vi "Read Aweight.vi"(8 "error in (no error)":errorcluster, 11 "Noise in":refnum<class "Noise.lvclass">) -> (0 "error out":errorcluster, 2 "Aweight":bool, 3 "Noise out":refnum<class "Noise.lvclass">)   [LabVIEW 2020, in "Noise.lvclass"]
uses:
  Noise.lvclass
  Noise.lvclass/Noise.ctl
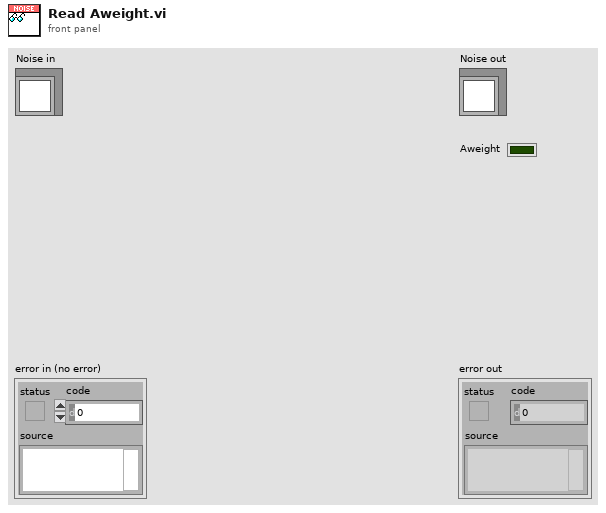
[diagram p1: front panel]
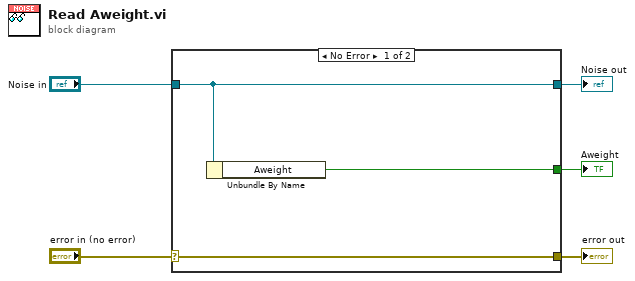
[diagram p0: block diagram]
diagram:
  n1 = case shown="No Error" "error in (no error)" {
    selector: "error in (no error)" -> [w8 w9]
    tunnel: [w8 w9] -> w4
    tunnel: [w7 w10] -> w2
    tunnel: "Noise in" -> [w7 w10]
    tunnel: [w6 _] -> w1
    frame No Error {
      n2 = Unbundle By Name(w7) -> ("Aweight"=w6:bool)
    }
    frame Error {
    }
  }
  "error out" <- w4
  "Noise out" <- w2
  "Aweight" <- w1
